vi "MassFlowDerivative.vi"(11 "Dynamic Data":dynamicdata(waveform)) -> (3 "Filtered x":dbl)   [LabVIEW 2020]
uses:
  <vilib>/ptbypt/NI_PtbyPt.lvlib
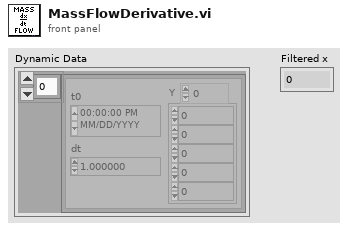
[diagram p1: front panel]
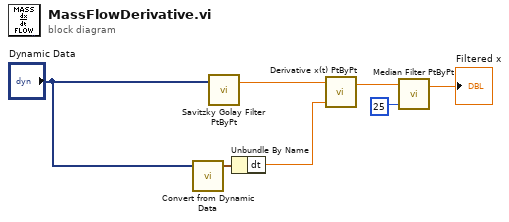
[diagram p0: block diagram]
diagram:
  n1 = call "Convert from Dynamic Data"("Dynamic Data Type"="Dynamic Data") -> ("Waveform"=w2:waveform(dbl))  [unwired: 3 in]
  n2 = call <vilib>:"Savitzky Golay Filter PtByPt.vi"("x"="Dynamic Data") -> ("Filtered x"=w1:dbl)  [unwired: 3 in, 1 out]
  n3 = Unbundle By Name(w2) -> ("dt"=w3:dbl)
  n4 = call <vilib>:"Derivative x(t) PtByPt.vi"("dt"=w3, "x"=w1) -> ("dx/dt"=w4:dbl)  [unwired: 2 in, 1 out]
  n5 = call <vilib>:"Median Filter PtByPt.vi"("rank"=25, "x"=w4) -> ("Filtered x"=→"Filtered x":dbl)  [unwired: 2 in, 1 out]
